vi "car arrows.vi"(0 "A PW1 duty":dbl=0.5, 1 "A PW1   ref":T1, 3 "A PW 2 ref":T1, 5 "A PW 2 duty":dbl=0.5, 7 "B PW1 duty":dbl=0.5, 9 "B PW2 duty":dbl=0.5, 11 "error in (no error)":errorcluster, 12 "B PW1 ref":T1, 14 "B PW2 ref":T1) -> (4 "PWM Ref Out":T1, 6 "PWM Ref Out 2":T1, 8 "PWM Ref Out 3":T1, 10 "PWM Ref Out 4":T1, 15 "error IO":errorcluster)   [LabVIEW 2016]
uses:
  <vilib>/myRIO/Instrument Drivers/Onboard IO/PWM/typedefs/PWM Reference.ctl
  <vilib>/myRIO/Common/Instrument Driver Framework/Utilities/typedefs/myRIO Generic Hardware Reference.ctl
  <vilib>/myRIO/Common/Instrument Driver Framework/Utilities/typedefs/Hardware Version Enum.ctl
  <vilib>/myRIO/Common/Instrument Driver Framework/Utilities/typedefs/myRIO v1.0 Reference.ctl
  <vilib>/myRIO/Common/Instrument Driver Framework/Utilities/typedefs/Generic FPGA Reference.ctl
  <vilib>/myRIO/Common/Instrument Driver Framework/myRIO v1.0/PWM/typedefs/PWM Channels Enum.ctl
  <vilib>/myRIO/Instrument Drivers/Onboard IO/PWM/typedefs/PWM Configuration.ctl
  <vilib>/myRIO/Instrument Drivers/Onboard IO/PWM/vis/Set Duty Cycle and Frequency.vi
  <vilib>/Utility/error.llb/Error Cluster From Error Code.vi
  <vilib>/myRIO/Common/Instrument Driver Framework/myRIO v1.0/PWM/vis/myRIO v1.0 Write PWM.vi
  <vilib>/ErrorRing/Error Ring.xnode
  <vilib>/myRIO/Instrument Drivers/Onboard IO/PWM/PWM.lvlib
panel:
  # "A PW 2"
  # "A PW 1"
  # "B PW 1"
  # "B PW 2"
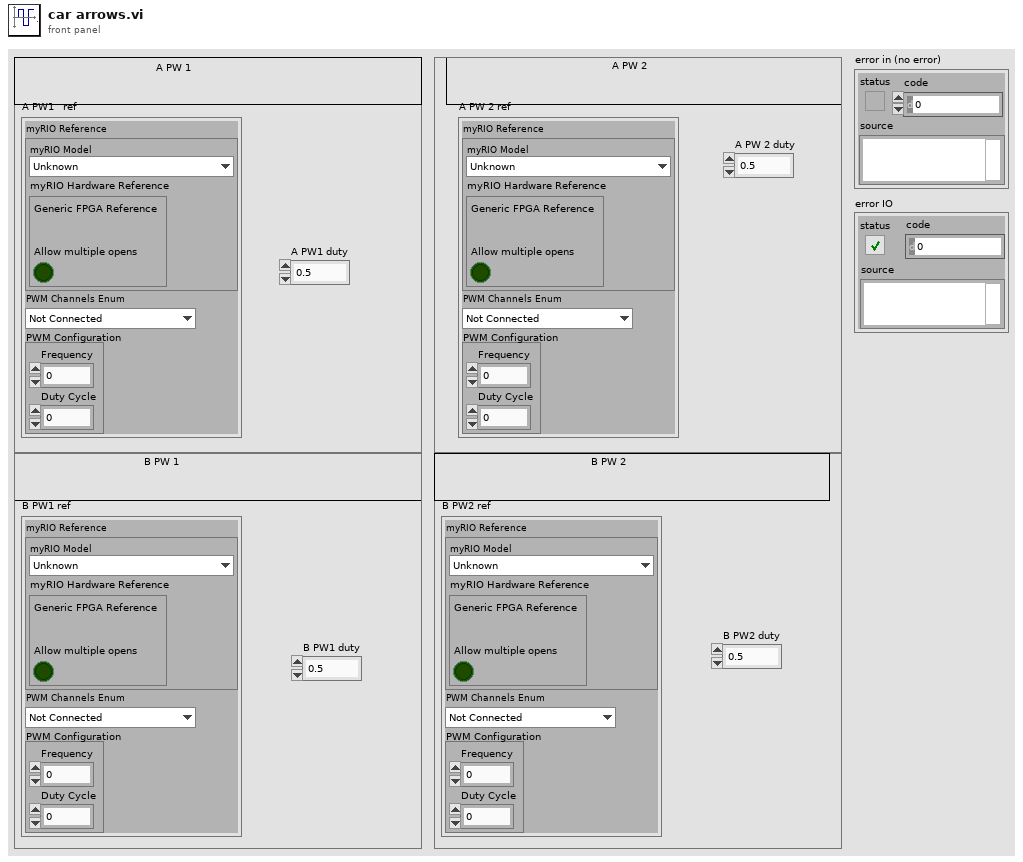
[diagram p1: front panel]
types:
  T1 = typedef "PWM.lvlib/PWM Reference.ctl" = cluster{"myRIO Reference":T2, "PWM Channels Enum":T6, "PWM Configuration":T7}
  T2 = typedef "myRIO Generic Hardware Reference.ctl" = cluster{"myRIO Model":T3, "myRIO Hardware Reference":T4}
  T3 = typedef "Hardware Version Enum.ctl" = enum16{"Unknown", "myRIO-1900", "myRIO-1950", "roboRIO", "NI ELVIS RIO CM"}
  T4 = typedef "myRIO v1.0 Reference.ctl" = cluster{"Generic FPGA Reference":T5, "Allow multiple opens":bool}
  T5 = typedef "Generic FPGA Reference.ctl" = refnum<k20>
  T6 = typedef "PWM Channels Enum.ctl" = enum16{"Not Connected", "C/PWM0", "C/PWM1", "A/PWM0", "A/PWM1", "A/PWM2", "B/PWM0", "B/PWM1", "B/PWM2", "PWM/PWM0", "PWM/PWM1", "PWM/PWM2", "PWM/PWM3", "PWM/PWM4", "PWM/PWM5", "PWM/PWM6", "PWM/PWM7", "PWM/PWM8", "PWM/PWM9"}
  T7 = typedef "PWM.lvlib/PWM Configuration.ctl" = cluster{"Frequency":dbl, "Duty Cycle":dbl}
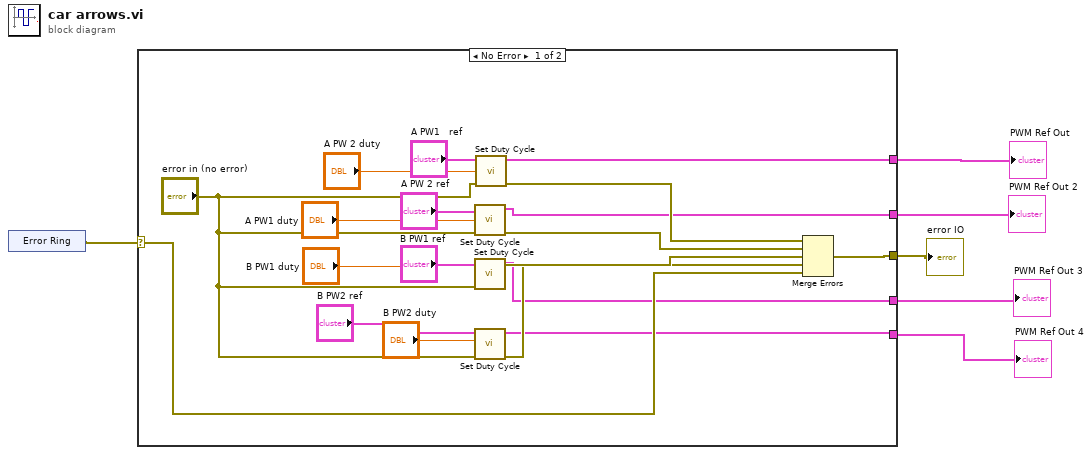
[diagram p0: block diagram]
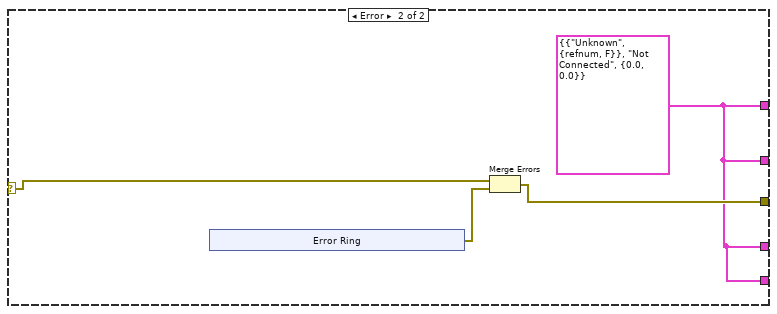
[diagram p2: hidden frame]
diagram:
  n1 = xnode "Error Ring"() -> ("error out"=w6:errorcluster)
  n2 = case shown="No Error" w6 {
    selector: w6 -> [w12 w29]
    tunnel: [w11 w27] -> w5
    tunnel: [w10 w26] -> w4
    tunnel: [w9 w26] -> w3
    tunnel: [w8 w26] -> w2
    tunnel: [w7 w26] -> w1
    frame No Error {
      n3 = call <vilib>:"Set Duty Cycle.vi"("error in (no error)"="error in (no error)", "Duty Cycle"="A PW1 duty", "PWM Ref In"="A PW 2 ref") -> ("error out"=w15:errorcluster, "PWM Ref Out"=w9:T1)  [unwired: 6 in]
      n4 = call <vilib>:"Set Duty Cycle.vi"("error in (no error)"="error in (no error)", "Duty Cycle"="B PW1 duty", "PWM Ref In"="B PW1 ref") -> ("error out"=w14:errorcluster, "PWM Ref Out"=w8:T1)  [unwired: 6 in]
      n5 = call <vilib>:"Set Duty Cycle.vi"("error in (no error)"="error in (no error)", "Duty Cycle"="B PW2 duty", "PWM Ref In"="B PW2 ref") -> ("error out"=w13:errorcluster, "PWM Ref Out"=w7:T1)  [unwired: 6 in]
      n6 = call <vilib>:"Set Duty Cycle.vi"("error in (no error)"="error in (no error)", "Duty Cycle"="A PW 2 duty", "PWM Ref In"="A PW1   ref") -> ("error out"=w16:errorcluster, "PWM Ref Out"=w10:T1)  [unwired: 6 in]
      n7 = Merge Errors(w16, w15, w14, w13, w12) -> (w11:errorcluster)
    }
    frame Error {
      w26 = T1 {"myRIO Reference"={"myRIO Model"=enum."Unknown", "myRIO Hardware Reference"={"Generic FPGA Reference"=refnum, "Allow multiple opens"=FALSE}}, "PWM Channels Enum"=enum."Not Connected", "PWM Configuration"={"Frequency"=0.0, "Duty Cycle"=0.0}} ("PWM Ref Out")
      n8 = xnode "Error Ring"() -> ("error out"=w28:errorcluster)
      n9 = Merge Errors(w29, w28) -> (w27:errorcluster)
    }
  }
  "error IO" <- w5
  "PWM Ref Out" <- w4
  "PWM Ref Out 2" <- w3
  "PWM Ref Out 3" <- w2
  "PWM Ref Out 4" <- w1
